vi "Initialize Manifold.vi"(8 "error in":errorcluster, 11 "Gantry in":refnum<class "Gantry.lvclass">) -> (0 "error out":errorcluster, 3 "Gantry out":refnum<class "Gantry.lvclass">)   [LabVIEW 2026, in "Gantry.lvclass"]
uses:
  Gantry.lvclass
  <vilib>/DAQmx/miscellaneous.llb/DAQmx Fill In Error Info.vi
  FlexWorktable/FlexWorktable.lvclass
  Gantry.lvclass/Gantry.ctl
  <vilib>/DAQmx/create/channels.llb/DAQmx Create Channel (DO-Digital Output).vi
  <vilib>/DAQmx/write.llb/DAQmx Write (Digital 1D Bool NChan 1Samp 1Line).vi
  GH2/GH2.lvclass
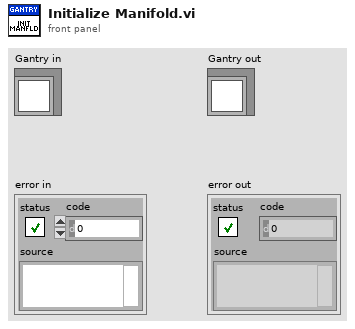
[diagram p1: front panel]
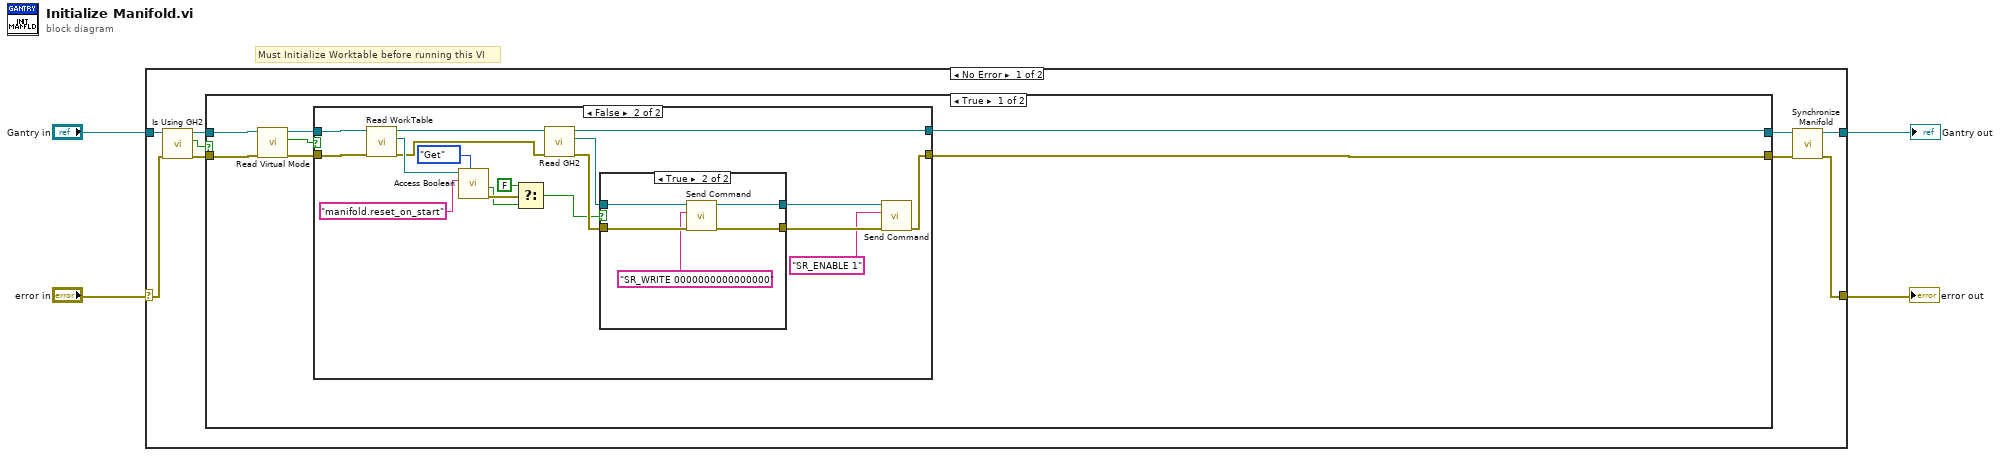
[diagram p0: block diagram]
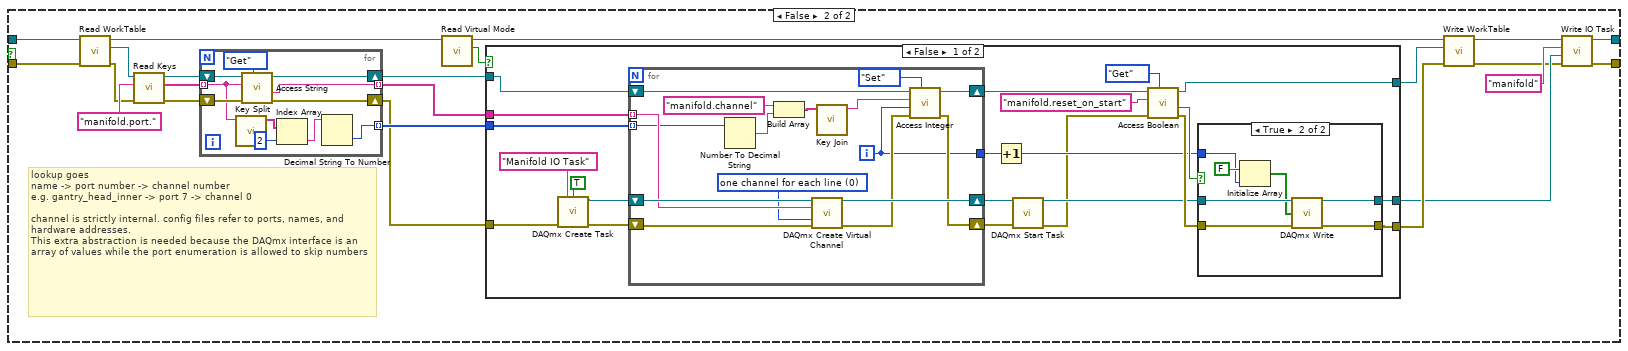
[diagram p4: hidden frame]
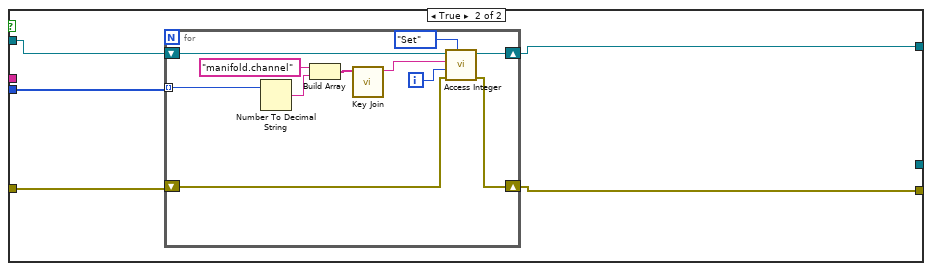
[diagram p6: hidden frame]
diagram:
  # "Must Initialize Worktable before running this VI"
  n1 = case shown="No Error" "error in" {
    selector: "error in" -> [w7 w146]
    tunnel: [w12 w146] -> w2
    tunnel: [w13 w145] -> w1
    tunnel: "Gantry in" -> [w9 w145]
    frame No Error {
      n2 = call "Is Using GH2.vi"("error in (no error)"=w7, "Gantry in"=w9) -> ("error out"=w6:errorcluster, "Using GH2"=w5:bool, "Gantry out"=w8:refnum<class "Gantry.lvclass">)  [unwired: 7 in]
      n3 = case shown="True" w5 {
        tunnel: [w20 w70] -> w11
        tunnel: [w19 w68] -> w10
        tunnel: w8 -> [w18 w52]
        tunnel: w6 -> [w16 w51]
        frame True {
          n4 = call-dynamic "Read Virtual Mode.vi"("error in (no error)"=w16, "Gantry in"=w18) -> ("error out"=w15:errorcluster, "Is Virtual"=w14:bool, "Gantry out"=w17:refnum<class "Gantry.lvclass">)  [unwired: 6 in, 1 out]
          n5 = case shown="False" w14 {
            tunnel: [w22 w26] -> w20
            tunnel: [w21 w25] -> w19
            tunnel: w17 -> [w22 w24]
            tunnel: w15 -> [w21 w23]
            frame True {
            }
            frame False {
              n6 = call-dynamic "Read WorkTable.vi"("error in"=w23, "Gantry Class in"=w24) -> ("error out"=w32:errorcluster, "Worktable"=w38:refnum<class "FlexWorktable.lvclass">, "Gantry Class out"=w37:refnum<class "Gantry.lvclass">)  [unwired: 7 in]
              n7 = call-dynamic "Access Boolean.vi"("Get/Set"=enum16{"Get", "Set"}."Get", "Key"="manifold.reset_on_start" ("Label"), "FlexWorktable in"=w38) -> ("error out"=w34:errorcluster, "Value out"=w33:bool)  [unwired: 6 in, 1 out]
              n8 = Select(t=FALSE, s=w34, f=w33) -> (s? t:f=w30:bool)
              n9 = call "Read GH2.vi"("error in (no error)"=w32, "Gantry in"=w37) -> ("error out"=w35:errorcluster, "GH2.lvclass"=w36:refnum<class "GH2.lvclass">, "Gantry out"=w26:refnum<class "Gantry.lvclass">)  [unwired: 7 in]
              n10 = case shown="True" w30 {
                tunnel: w36 -> [w42 w47]
                tunnel: w35 -> [w41 w46]
                tunnel: [w42 w44] -> w29
                tunnel: [w41 w43] -> w28
                frame False {
                }
                frame True {
                  n11 = call "Send Command.vi"("error in (no error)"=w46, "command"="SR_WRITE 0000000000000000", "GH2 in"=w47) -> ("error out"=w43:errorcluster, "GH2 out"=w44:refnum<class "GH2.lvclass">)  [unwired: 6 in, 1 out]
                }
              }
              n12 = call "Send Command.vi"("error in (no error)"=w28, "command"="SR_ENABLE 1", "GH2 in"=w29) -> ("error out"=w25:errorcluster)  [unwired: 6 in, 2 out]
            }
          }
        }
        frame False {
          # "lookup goes\nname -> port number -> channel number\ne.g. gantry_head_inner -> port 7 -> channel 0\n\nchannel is strictly internal. config files refer to ports, names, and hardware addresses.\nThis extra abstraction is needed because the DAQmx interface is an array of values while the port enumeration is allowed to skip numbers"
          n13 = call-dynamic "Read WorkTable.vi"("error in"=w51, "Gantry Class in"=w52) -> ("error out"=w65:errorcluster, "Worktable"=w67:refnum<class "FlexWorktable.lvclass">, "Gantry Class out"=w50:refnum<class "Gantry.lvclass">)  [unwired: 7 in]
          n14 = call-dynamic "Read Keys.vi"("error in (no error)"=w65, "Selector"="manifold.port.", "FlexWorktable in"=w67) -> ("error out"=w62:errorcluster, "Keys"=w63:string[], "FlexWorktable out"=w64:refnum<class "FlexWorktable.lvclass">)  [unwired: 6 in]
          n15 = for {
            tunnel: [w77] -> w61 mode=indexing
            tunnel: w63 -> [w75] mode=indexing
            shift-right: [w80] -> w59
            shift-left: w64 -> [w81]
            shift-right: [w78] -> w58
            shift-left: w62 -> [w79]
            tunnel: [w71] -> w60 mode=indexing
            n16 = call "Key Split.vi"("Key"=w75) -> ("Key Elements"=w74:string[])  [unwired: 10 in]
            n17 = call-dynamic "Access String.vi"("Get/Set"=enum16{"Get", "Set"}."Get", "error in (no error)"=w79, "Key"=w75, "FlexWorktable in"=w81) -> ("error out"=w78:errorcluster, "Value out"=w77:string, "FlexWorktable out"=w80:refnum<class "FlexWorktable.lvclass">)  [unwired: 5 in]
            n18 = Index Array(array=w74, index=2) -> (element=w72:string)
            n19 = Decimal String To Number(string=w72) -> (number=w71:i32)  [unwired: 2 in, 1 out]
          }
          n20 = call-dynamic "Read Virtual Mode.vi"("Gantry in"=w50) -> ("Is Virtual"=w48:bool, "Gantry out"=w49:refnum<class "Gantry.lvclass">)  [unwired: 7 in, 2 out]
          n21 = case shown="False" w48 {
            tunnel: w61 -> [w100 _]
            tunnel: w60 -> [w99 w132]
            tunnel: w59 -> [w96 w133]
            tunnel: w58 -> [w101 w131]
            tunnel: [w84 w129] -> w55
            tunnel: [w83 w130] -> w56
            tunnel: [w82 _] -> w54
            frame False {
              n22 = call <vilib>:"DAQmx Create Task.vi"("new task name"="Manifold IO Task", "auto cleanup"=TRUE, "error in"=w101) -> ("task out"=w98:refnum<k21>, "error out"=w97:errorcluster)  [unwired: 2 in, 9 out]
              n23 = for {
                tunnel: w100 -> [w126] mode=indexing
                tunnel: w99 -> [w114] mode=indexing
                shift-right: [w127] -> w88
                shift-left: w98 -> [w128]
                shift-right: [w120] -> w86
                shift-left: w97 -> [w125]
                shift-right: [w119] -> w93
                shift-left: w96 -> [w123]
                tunnel: [w113] -> w90
                i -> [w113]
                w124 = 0 items=["one channel for each line", "one channel for all lines"] ("line grouping")
                n24 = Number To Decimal String(number=w114) -> (decimal integer string=w115:string)  [unwired: 1 in]
                n25 = Build Array("manifold.channel", w115) -> (w117:string[])
                n26 = call-poly <vilib>:"DAQmx Create Virtual Channel.vi"("task in"=w128, "lines"=w126, "line grouping"=w124, "error in"=w125) -> ("task out"=w127:refnum<k21>, "error out"=w121:errorcluster)  [unwired: 1 in, 9 out]
                n27 = call "Key Join.vi"("Key Elements"=w117) -> ("Key"=w118:string)  [unwired: 10 in]
                n28 = call-dynamic "Access Integer.vi"("Get/Set"=enum16{"Get", "Set"}."Set", "error in (no error)"=w121, "Value in"=w113, "Key"=w118, "FlexWorktable in"=w123) -> ("error out"=w120:errorcluster, "FlexWorktable out"=w119:refnum<class "FlexWorktable.lvclass">)  [unwired: 4 in, 1 out]
              }
              n29 = Increment(x=w90) -> (x+1=w89:i32)
              n30 = call <vilib>:"DAQmx Start Task.vi"("task/channels in"=w88, "error in"=w86) -> ("task out"=w87:refnum<k21>, "error out"=w85:errorcluster)  [unwired: 12 out]
              n31 = call-dynamic "Access Boolean.vi"("Get/Set"=enum16{"Get", "Set"}."Get", "error in (no error)"=w85, "Key"="manifold.reset_on_start" ("Label"), "FlexWorktable in"=w93) -> ("error out"=w91:errorcluster, "Value out"=w92:bool, "FlexWorktable out"=w84:refnum<class "FlexWorktable.lvclass">)  [unwired: 5 in]
              n32 = case shown="True" w92 {
                tunnel: w91 -> [w104 w112]
                tunnel: w87 -> [w105 w111]
                tunnel: w89 -> [_ w109]
                tunnel: [w105 w107] -> w82
                tunnel: [w104 w106] -> w83
                frame False {
                }
                frame True {
                  n33 = Initialize Array(FALSE, w109) -> (w108:bool[])
                  n34 = call-poly <vilib>:"DAQmx Write.vi"("task/channels in"=w111, "data"=w108, "error in"=w112) -> ("task out"=w107:refnum<k21>, "error out"=w106:errorcluster)  [unwired: 10 in, 1 out]
                }
              }
            }
            frame True {
              n35 = for {
                tunnel: w132 -> [w136] mode=indexing
                shift-right: [w142] -> w130
                shift-left: w131 -> [w135]
                shift-right: [w141] -> w129
                shift-left: w133 -> [w144]
                i -> [w134]
                n36 = Number To Decimal String(number=w136) -> (decimal integer string=w137:string)  [unwired: 1 in]
                n37 = Build Array("manifold.channel", w137) -> (w139:string[])
                n38 = call "Key Join.vi"("Key Elements"=w139) -> ("Key"=w140:string)  [unwired: 10 in]
                n39 = call-dynamic "Access Integer.vi"("Get/Set"=enum16{"Get", "Set"}."Set", "error in (no error)"=w135, "Value in"=w134, "Key"=w140, "FlexWorktable in"=w144) -> ("error out"=w142:errorcluster, "FlexWorktable out"=w141:refnum<class "FlexWorktable.lvclass">)  [unwired: 4 in, 1 out]
              }
            }
          }
          n40 = call-dynamic "Write WorkTable.vi"("error in (no error)"=w56, "FlexWorktable"=w55, "Gantry Class in"=w49) -> ("error out"=w53:errorcluster, "Gantry Class out"=w57:refnum<class "Gantry.lvclass">)  [unwired: 7 in]
          n41 = call "Write IO Task.vi"("error in (no error)"=w53, "IO Task"=w54, "Task Name"="manifold", "Gantry in"=w57) -> ("error out"=w68:errorcluster, "Gantry out"=w70:refnum<class "Gantry.lvclass">)  [unwired: 6 in]
        }
      }
      n42 = call-dynamic "Synchronize Manifold.vi"("error in"=w10, "Gantry in"=w11) -> ("error out"=w12:errorcluster, "Gantry out"=w13:refnum<class "Gantry.lvclass">)  [unwired: 8 in]
    }
    frame Error {
    }
  }
  "error out" <- w2
  "Gantry out" <- w1
